vi "HomeCMD.vi"(8 "Error In":errorcluster, 11 "Thorlabs In":refnum<class "Thorlabs.lvclass">) -> (0 "Error Out":errorcluster, 3 "Thorlabs Out":refnum<class "Thorlabs.lvclass">)   [LabVIEW 2018, in "Thorlabs.lvlib" / "Thorlabs.lvclass"]
doc: "This vi tells the Device to go Home. Since we don't want this to block, it sends the CMD but does not verify that it was finished. Call Parse Respond Message and then Read Response to verify whether it completed or not.\n\nCreator: Slade Jeppesen\nCreated Date: 09/29/20"
uses:
  Thorlabs.lvclass
  Thorlabs.lvclass/Thorlabs.ctl
  C:/AME Test Engineering/LabVIEW/PPLs/Axis/DLLs/ThorLabs.MotionControl.KCube.DCServoCLI.dll
  PPLs/Axis/DLLs/ThorLabs.MotionControl.KCube.DCServoCLI.dll
  cb28d17c-625b-4aa2-a1e6-dd2d5a3da7f7.vi
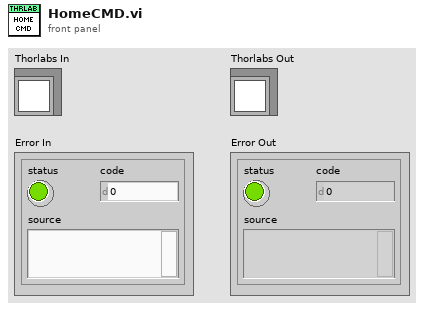
[diagram p1: front panel]
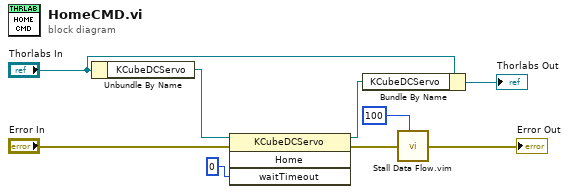
[diagram p0: block diagram]
diagram:
  n1 = Unbundle By Name("Thorlabs In") -> ("KCubeDCServo"=w6:refnum<k24>)
  n2 = invoke class="KCubeDCServo" method="Home"(reference=w6, error in="Error In", "waitTimeout"=0) -> (reference out=w7:refnum<k24>, error out=w3:errorcluster)  [unwired: 1 in, 2 out]
  n3 = Bundle By Name(cluster="Thorlabs In", "KCubeDCServo"=w7) -> (→"Thorlabs Out":refnum<class "Thorlabs.lvclass">)
  n4 = call "Stall Data Flow.vim"("value in"=w3, "milliseconds to wait"=u32 100) -> ("value out"=→"Error Out":errorcluster)  [unwired: 1 out]
